vi "Create Data File - Config.vi"(8 "error in (no error)":errorcluster, 10 "Acquisition Data v1":T1={"Data Rate"=1, "Samples per Read"=0, "Number of Reads to Save"=0, "Data File Name"="", "TDMS Properties"=[], "Number of Channels"=4, "Channel Scale Array"=[0.0, 0.0, 0.0, 0.0, 0.0, 0.0, 0.0, 0.0, 0.0, 0.0, 0.0, 0.0, 0.0, 0.0, 0.0, 0.0, 0.0, 0.0, 0.0, 0.0, 0.0, 0.0, 0.0, 0.0], "Channel Names"=[], "Trigger - RMS Value"=0.0, "Trigger - Channel"=0, "Trigger - Time (Minute)"=0, "Input Configuration Array"=[]} {"Input Configuration Array" items=["AC Coupled", "DC Coupled", "IEPE AC Coupled"]; "Data Rate" items=["51.200 kS/s (NI 9234)"=1, "25.600 kS/s (NI 9234)"=2, "17.067 kS/s (NI 9234)"=3, "12.800 kS/s (NI 9234)"=4, "10.240 kS/s (NI 9234)"=5, "8.533 kS/s (NI 9234)"=6, "7.314 kS/s (NI 9234)"=7, "6.400 kS/s (NI 9234)"=8, "5.689 kS/s (NI 9234)"=9, "5.120 kS/s (NI 9234)"=10, "4.654 kS/s (NI 9234)"=11, "4.267 kS/s (NI 9234)"=12, "3.938 kS/s (NI 9234)"=13, "3.657 kS/s (NI 9234)"=14, "3.413 kS/s (NI 9234)"=15, "3.200 kS/s (NI 9234)"=16, "3.012 kS/s (NI 9234)"=17, "2.845 kS/s (NI 9234)"=18, "2.695 kS/s (NI 9234)"=19, "2.560 kS/s (NI 9234)"=20, "2.438 kS/s (NI 9234)"=21, "2.328 kS/s (NI 9234)"=22, "2.226 kS/s (NI 9234)"=23, "2.133 kS/s (NI 9234)"=24, "2.048 kS/s (NI 9234)"=25, "1.969 kS/s (NI 9234)"=26, "1.896 kS/s (NI 9234)"=27, "1.829 kS/s (NI 9234)"=28, "1.765 kS/s (NI 9234)"=29, "1.707 kS/s (NI 9234)"=30, "1.652 kS/s (NI 9234)"=31]}) -> (0 "error out":errorcluster, 3 "TDMS File Reference":refnum<k34>)   [LabVIEW 2015]
doc: "Reads waveform data from the DMA FIFO."
uses:
  controls/Acquisition and Logging Configuration_v1.ctl
  <vilib>/LabVIEW Targets/FPGA/cRIO/shared/nicrio_ModuleControls/nicrio_cRIO-9234_DataRatesRing2.ctl
  controls/TDMS Properties.ctl
  <vilib>/LabVIEW Targets/FPGA/cRIO/shared/nicrio_ModuleControls/nicrio_cRIO-9234_ConfigModeRing.ctl
  Globals/Global - Configuration Options.vi
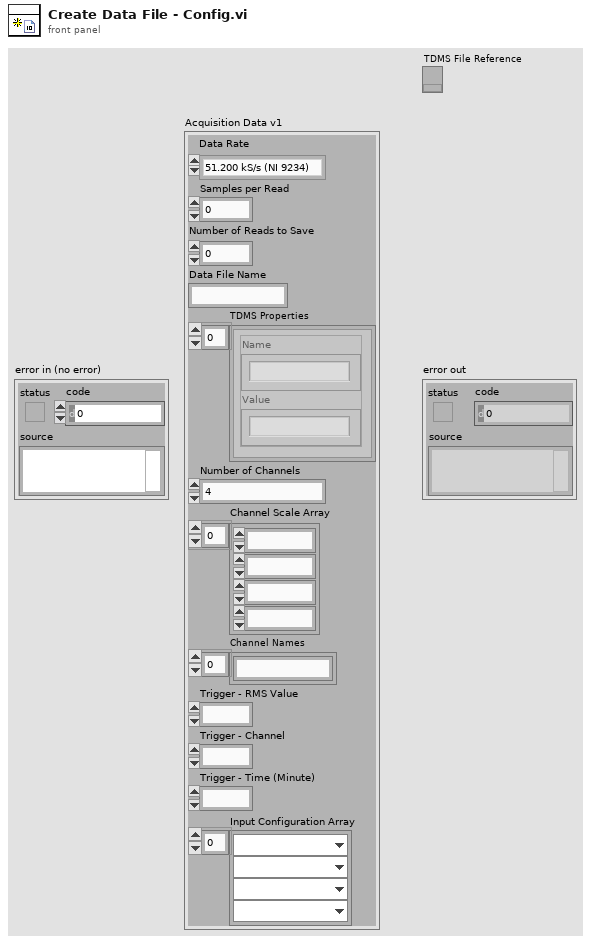
[diagram p1: front panel]
types:
  T1 = typedef "Acquisition and Logging Configuration_v1.ctl" = cluster{"Data Rate":T2, "Samples per Read":i32, "Number of Reads to Save":i32, "Data File Name":string, "TDMS Properties":T3[], "Number of Channels":i32, "Channel Scale Array":fxp<+,24,12>[], "Channel Names":string[], "Trigger - RMS Value":dbl, "Trigger - Channel":i32, "Trigger - Time (Minute)":i32, "Input Configuration Array":T4[]}
  T2 = typedef "nicrio_cRIO-9234_DataRatesRing2.ctl" = u8
  T3 = typedef "TDMS Properties.ctl" = cluster{"Name":string, "Value":string}
  T4 = typedef "nicrio_cRIO-9234_ConfigModeRing.ctl" = u8
  T5 = enum16{"open", "open or create", "create or replace", "create", "open (read-only)"}
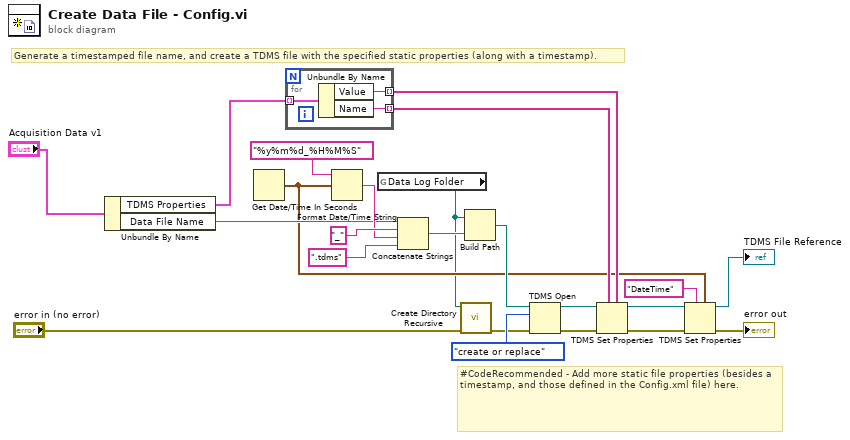
[diagram p0: block diagram]
diagram:
  # "Generate a timestamped file name, and create a TDMS file with the specified static properties (along with a timestamp)."
  # "#CodeRecommended - Add more static file properties (besides a timestamp, and those defined in the Config.xml file) here."
  n1 = Unbundle By Name("Acquisition Data v1") -> ("TDMS Properties"=w13:T3[], "Data File Name"=w19:string)
  n2 = Get Date/Time In Seconds() -> (seconds since 1Jan1904=w9:timestamp)
  n3 = for {
    tunnel: w13 -> [w26] mode=indexing
    tunnel: [w25] -> w12 mode=indexing
    tunnel: [w24] -> w11 mode=indexing
    n4 = Unbundle By Name(w26) -> ("Value"=w24:string, "Name"=w25:string)
  }
  n5 = Format Date/Time String(time format string (%c)="%y%m%d_%H%M%S", seconds (now)=w9) -> (date/time string=w22:string)  [unwired: 1 out]
  n6 = global read "Global - Configuration Options.vi" "Data Log Folder"() -> (w2:path)
  n7 = Concatenate Strings(w19, "_" ("string"), w22, ".tdms" ("string")) -> (w18:string)
  n8 = call <vilib>:"Create Directory Recursive.vi"("error in (no error)"="error in (no error)", "directory"=w2) -> ("error out"=w4:errorcluster)  [unwired: 3 in, 2 out]
  n9 = Build Path(base path=w2, name or relative path=w18) -> (appended path=w16:path)
  n10 = TDMS Open(8:w4, 10:T5."create or replace" ("operation (0:open)"), 11:w16) -> (0:w15:errorcluster, 3:w14:refnum<k34>)  [unwired: 4 in]
  n11 = TDMS Set Properties(5:w11, 7:w12, 8:w15, 11:w14) -> (0:w10:errorcluster, 3:w6:refnum<k34>)  [unwired: 2 in, 2 out]
  n12 = TDMS Set Properties(5:w9, 7:"DateTime" ("property names"), 8:w10, 11:w6) -> (0:→"error out":errorcluster, 3:→"TDMS File Reference":refnum<k34>)  [unwired: 2 in, 2 out]
